vi "Monitoring.vi"() -> ()   [LabVIEW 2014]
uses:
  <vilib>/Instr/_visa.llb/VISA Configure Serial Port (Instr).vi
  Downloads/AttitudeIndicator_lv2012/lv-attitudecontrol.lvlib
panel:
  in  "Tab Control":T1(tab)
  in  "Stop":bool
  in  "Connect":bool
  in  "VISA resource name":refnum<visa-resource-name>="ASRL1::INSTR"
  in  "baud rate":u32=115200
  in  "length of frame":u32=142
  out "error out":errorcluster
  in  "Afficher caractères reçus":bool
  out "received chars":string
  out "Serial Settings:Number of Bytes at Serial Port":u32
  out "Heading":i16
  out "Roll":i16
  out "Pitch":i16
  out "Roll":i16(graph)
  out "Pitch":i16(graph)
  out "Heading":i16(graph)
  in  "Attitude Indicator":refnum<vi>(3d-picture)
  out "Receiver":cluster{u16, u16, u16, u16, u16, u16, u16, u16}(graph)
  out "Ch 0":u16(slide) caption="Gear" scale=0.0..1000.0
  out "Throttle":u16(slide) scale=0.0..1000.0
  out "Roll":u16(slide) scale=0.0..1000.0
  out "Yaw":u16(slide) scale=0.0..1000.0
  out "Pitch":u16(slide) scale=0.0..1000.0
  out "Aux2":u16(slide) scale=0.0..1000.0
  out "Aux1":u16(slide) scale=0.0..1000.0
  out "N/D":u16(slide) scale=0.0..1000.0
  out "Armed":bool
  out "Motors":cluster{u16, u16, u16, u16, u16, u16, u16, u16}(graph)
  out "M 0":u16(slide) scale=0.0..1000.0
  out "M 7":u16(slide) scale=0.0..1000.0
  out "M 6":u16(slide) scale=0.0..1000.0
  out "M 5":u16(slide) scale=0.0..1000.0
  out "M 4":u16(slide) scale=0.0..1000.0
  out "M 3":u16(slide) scale=0.0..1000.0
  out "M 2":u16(slide) scale=0.0..1000.0
  out "M 1":u16(slide) scale=0.0..1000.0
  out "Servos":cluster{u16, u16, u16, u16}(graph)
  out "S 0":u16(slide) scale=0.0..1000.0
  out "S 3":u16(slide) scale=0.0..1000.0
  out "S 2":u16(slide) scale=0.0..1000.0
  out "S 1":u16(slide) scale=0.0..1000.0
  out "Meter":dbl(knob) scale=10800.0..12600.0
  out "Energy":u16
  out "Current":u16
  out "Voltage":u16
  out "Loop duration":u8
  out "Armed":bool
  out "SONAR 0":u16(slide) scale=0.0..1000.0
  out "BARO":u16(slide) scale=0.0..1000.0
  out "SONAR 5":u16(slide) scale=0.0..1000.0
  out "SONAR 4":u16(slide) scale=0.0..1000.0
  out "SONAR 3":u16(slide) scale=0.0..1000.0
  out "SONAR 2":u16(slide) scale=0.0..1000.0
  out "SONAR 1":u16(slide) scale=0.0..1000.0
  out "Baro":u16(graph)
  out "Sonars":cluster{u16, u16, u16, u16, u16, u16}(graph)
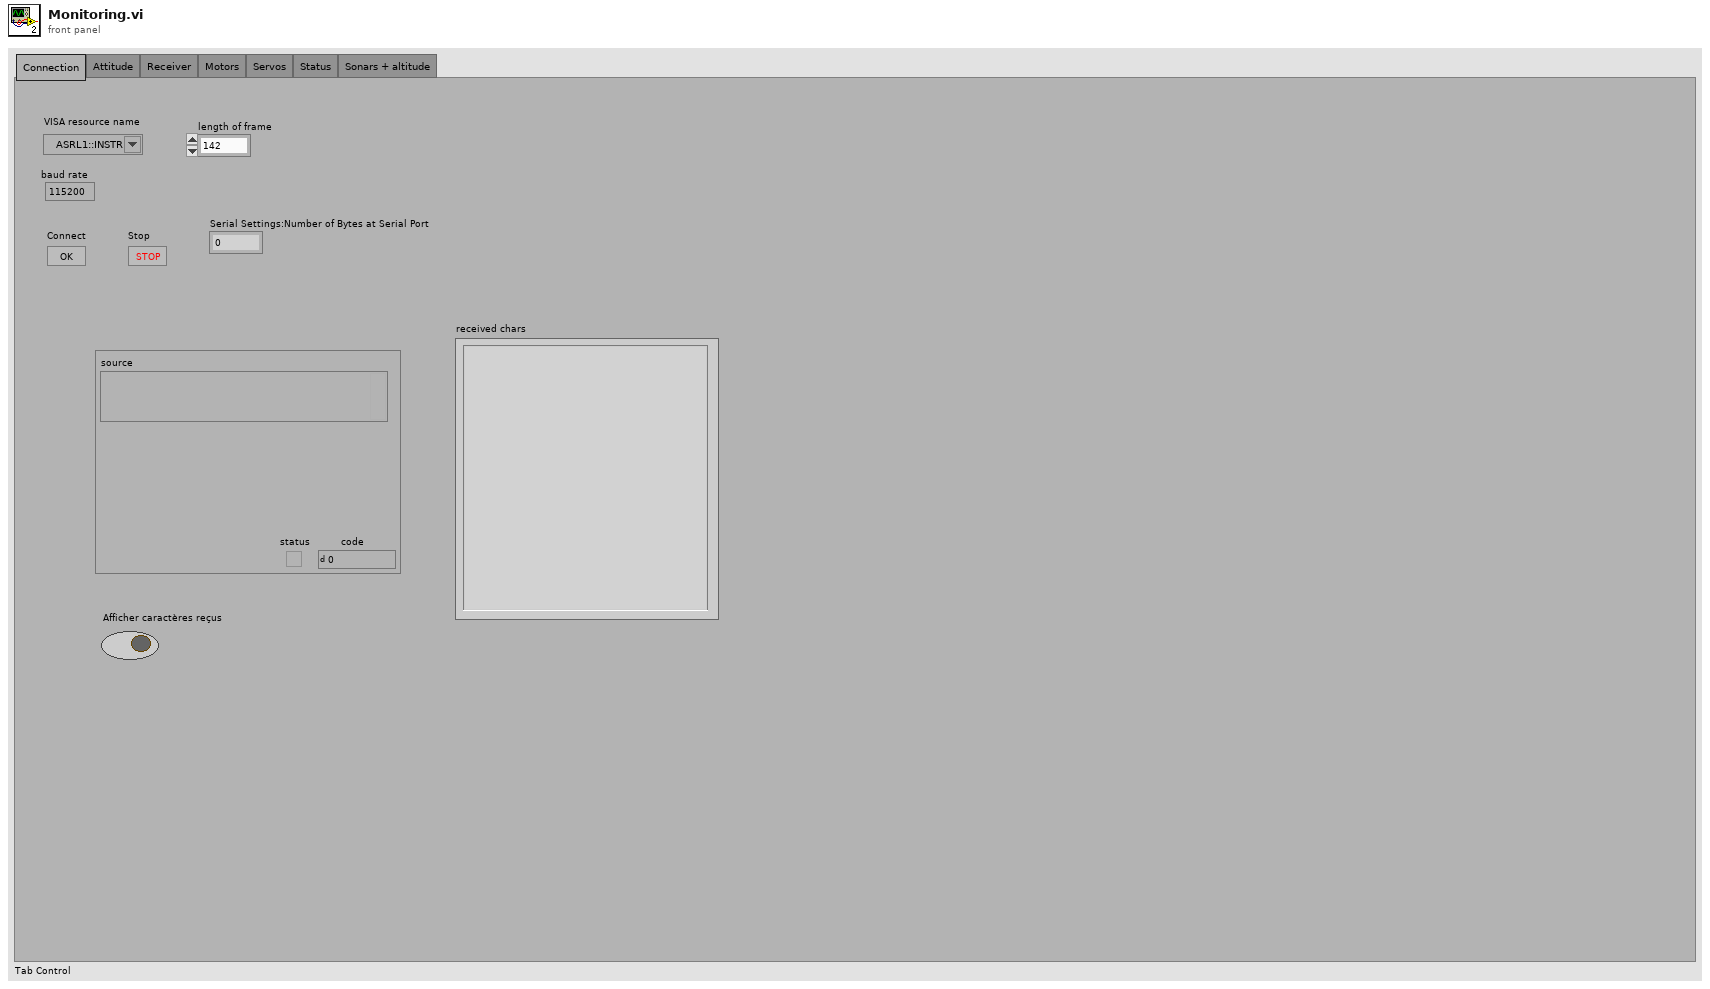
[diagram p1: front panel]
types:
  T1 = enum32{"Connection", "Attitude", "Receiver", "Motors", "Servos", "Status", "Sonars + altitude"}
  T2 = typedef "lv-attitudecontrol.lvlib/AttitudeHandle.ctl" = cluster{"First Scene Object":refnum<vi>, "Drum":refnum<vi>, "Window":refnum<vi>, "Dial":refnum<vi>, "Scene Graph":refnum<vi>, "Last Drum Pitch":dbl, "Last Drum Roll ":dbl, "Last Dial Roll":dbl}
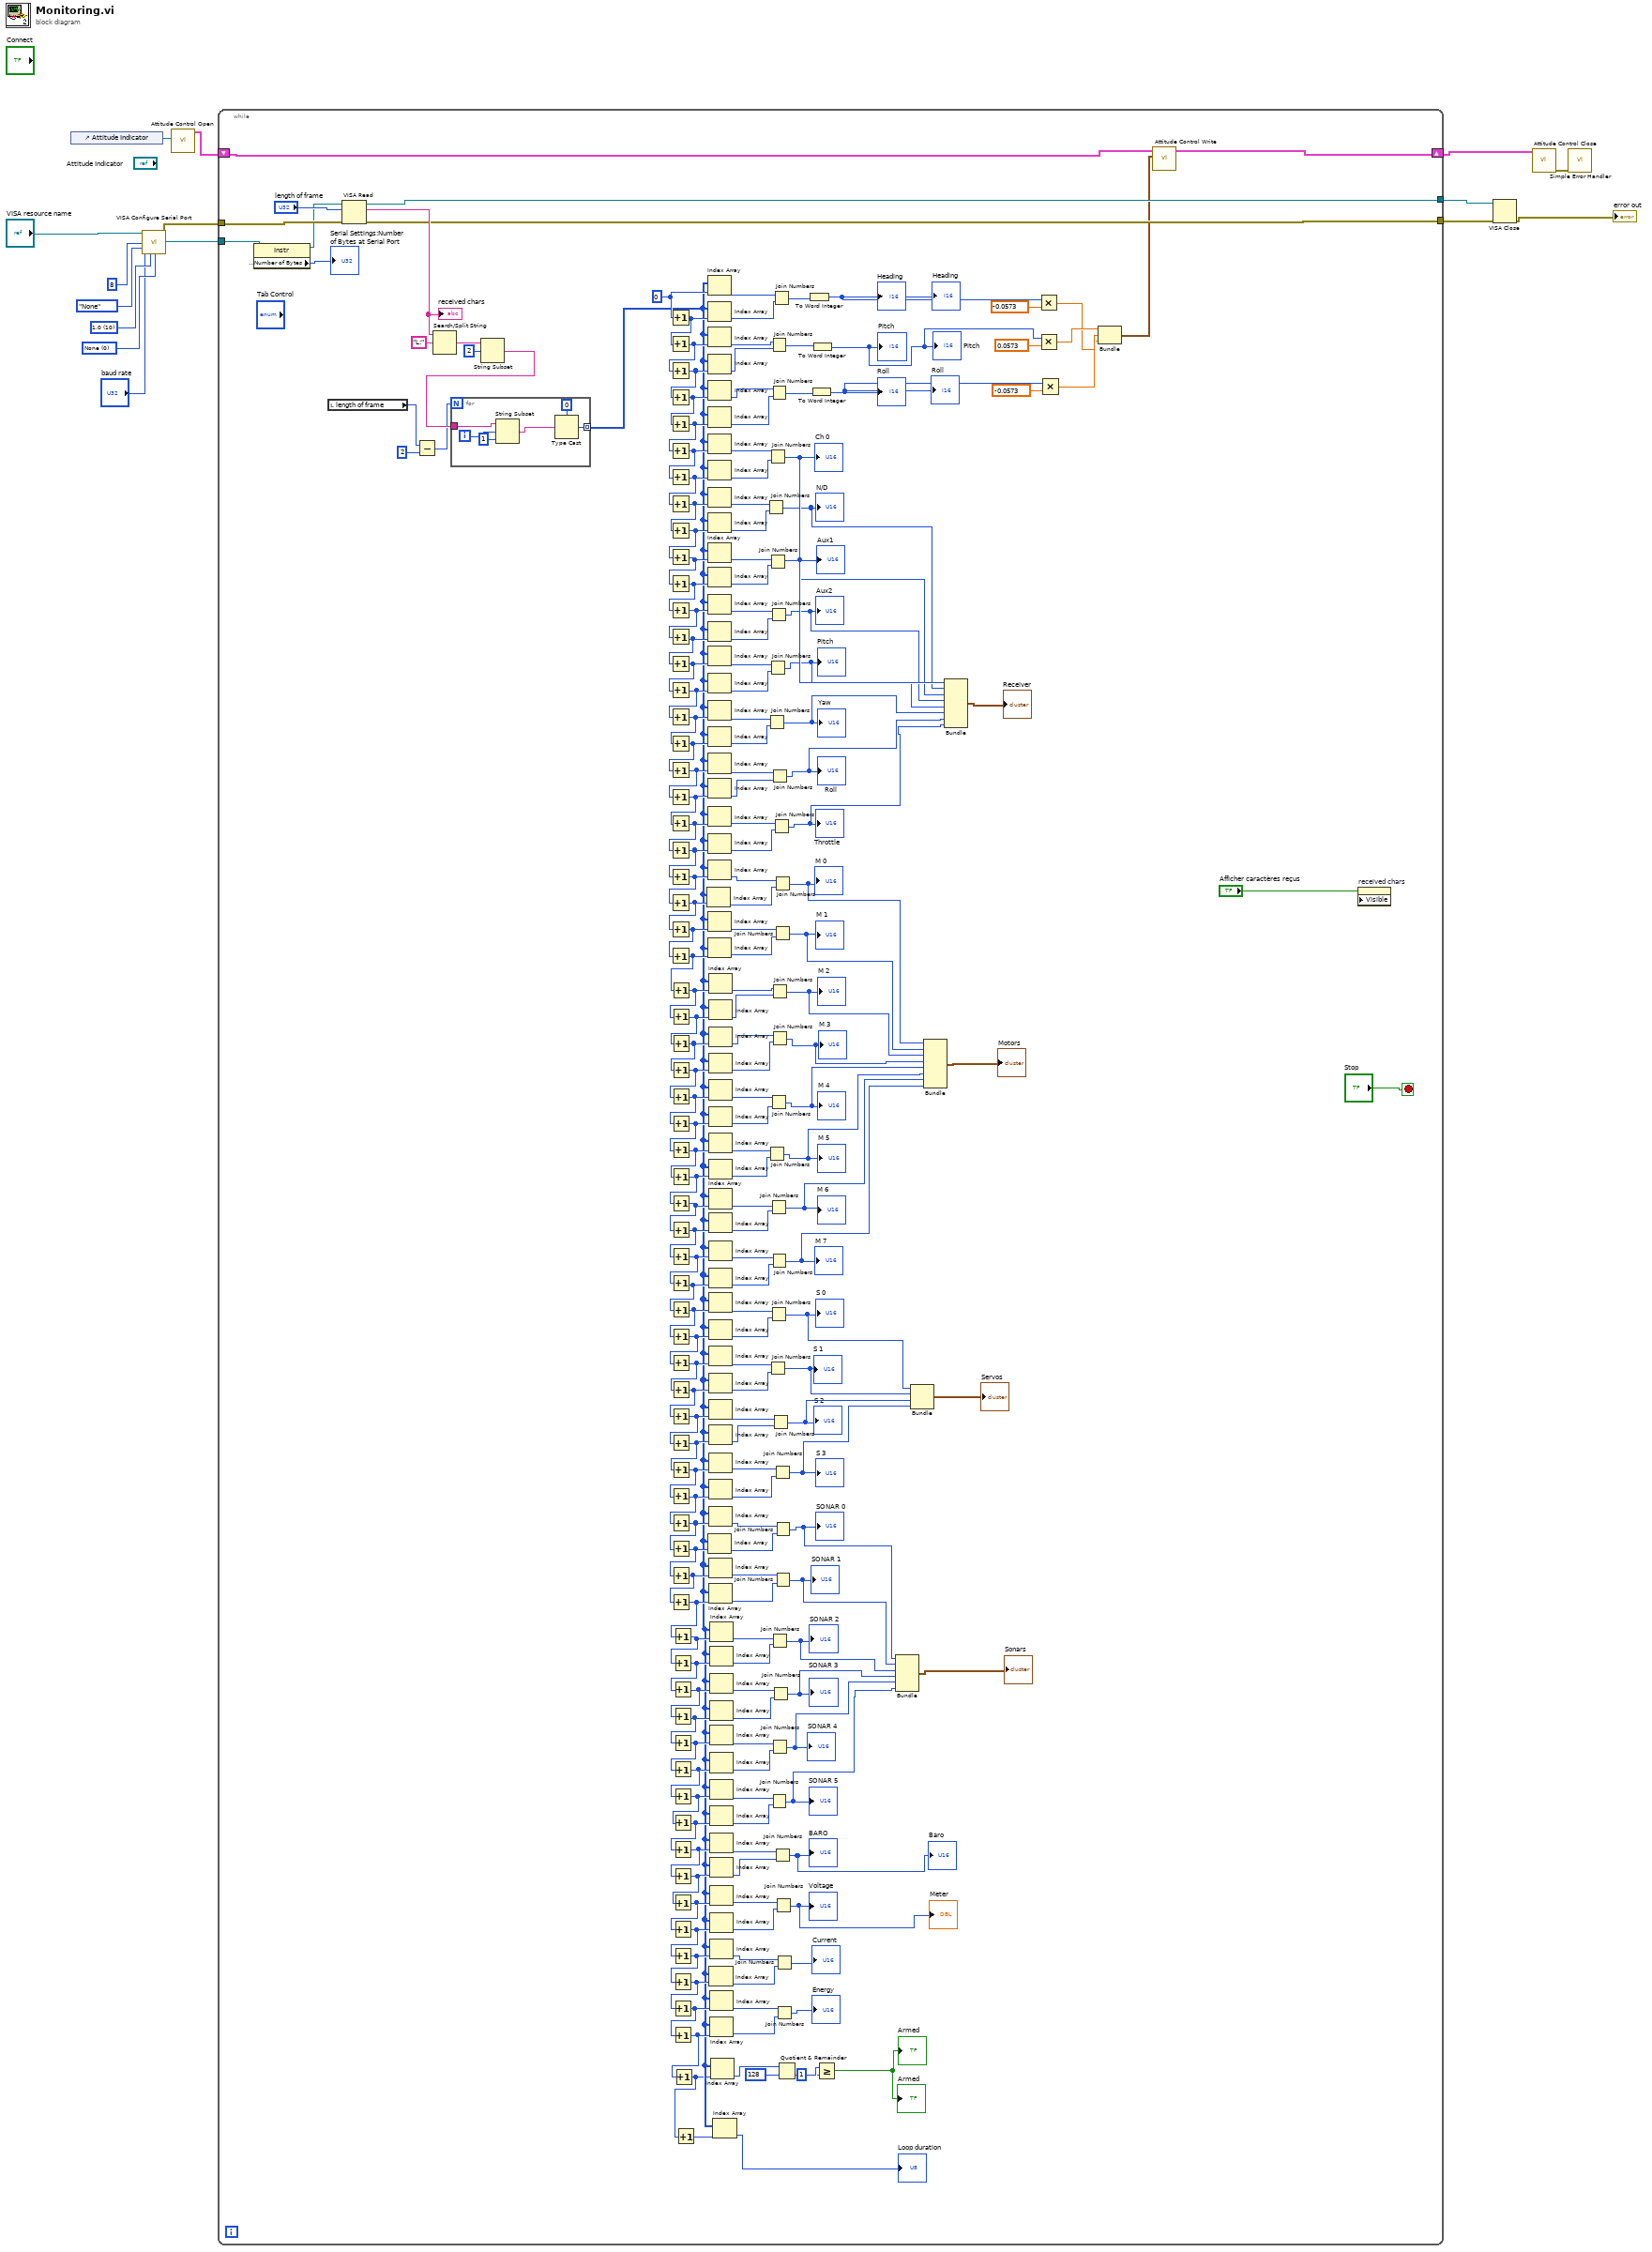
[diagram p0: block diagram]
diagram:
  w12 = u16 0 items=["None", "XON/XOFF", "RTS/CTS", "XON/XOFF & RTS/CTS", "DTR/DSR", "XON/XOFF & DTR/DSR"] ("flow control (0:none)")
  w13 = u16 10 items=["1.0"=10, "1.5"=15, "2.0"=20] ("stop bits (10: 1 bit)")
  n1 = control-ref of="Attitude Indicator"() -> (w4:refnum<vi>)
  n2 = call-poly "VISA Configure Serial Port"("VISA resource name"="VISA resource name", "baud rate (9600)"="baud rate", "data bits (8)"=u16 8, "parity (0:none)"=enum16{"None", "Odd", "Even", "Mark", "Space"}."None", "stop bits (10: 1 bit)"=w13, "flow control (0:none)"=w12) -> ("VISA resource name out"=w10:refnum<visa-resource-name>, "error out"=w9:errorcluster)  [unwired: 8 in]
  n3 = call "Attitude Control Open.vi"("Scene Graph"=w4) -> ("Attitude Control Handle"=w3:T2)  [unwired: 9 in, 1 out]
  n4 = while {
    tunnel: w10 -> [w40]
    tunnel: w9 -> [w192]
    tunnel: [w43] -> w7
    tunnel: [w41] -> w5
    shift-right: [w31] -> w1
    shift-left: w3 -> [w32]
    stop <- "Stop" stop-if-true
    w217 = 0 ("length")
    n5 = property class="Instr"(reference=w40) -> (reference out=w39:refnum<visa-resource-name>, "Serial Settings:Number of Bytes at Serial Port"=→"Serial Settings:Number of Bytes at Serial Port":u32)  [unwired: 1 in, 1 out]
    n6 = local read "length of frame"() -> (w35:u32)
    n7 = VISA Read(VISA resource name=w39, byte count="length of frame", error in (no error)=w192) -> (VISA resource name out=w41:refnum<visa-resource-name>, read buffer=w191:string, error out=w43:errorcluster)  [unwired: 1 out]
    "received chars" <- w191
    n8 = Subtract(x=w35, y=u32 2) -> (x-y=w33:u32)
    n9 = Search/Split String(string=w191, search string/char (-)="L:") -> (match + rest of string=w222:string)  [unwired: 1 in, 2 out]
    n10 = String Subset(string=w222, offset (0)=2) -> (substring=w218:string)  [unwired: 1 in]
    n11 = for {
      N: w33 -> [_]
      tunnel: w218 -> [w225]
      tunnel: [w224] -> w18 mode=indexing
      i -> [w223]
      n12 = String Subset(string=w225, offset (0)=w223, length (rest)=1 ("length (rest)")) -> (substring=w226:string)
      n13 = Type Cast(type=u8 0, x=w226) -> (*(type *) &x=w224:u8)
    }
    n14 = Increment(x=w217) -> (x+1=w216:i32)
    n15 = Increment(x=w216) -> (x+1=w215:i32)
    n16 = Increment(x=w215) -> (x+1=w214:i32)
    n17 = Increment(x=w214) -> (x+1=w213:i32)
    n18 = Increment(x=w213) -> (x+1=w212:i32)
    n19 = Increment(x=w212) -> (x+1=w211:i32)
    n20 = Increment(x=w211) -> (x+1=w210:i32)
    n21 = Increment(x=w210) -> (x+1=w209:i32)
    n22 = Increment(x=w209) -> (x+1=w208:i32)
    n23 = Increment(x=w208) -> (x+1=w207:i32)
    n24 = Increment(x=w207) -> (x+1=w206:i32)
    n25 = Increment(x=w206) -> (x+1=w205:i32)
    n26 = Increment(x=w205) -> (x+1=w204:i32)
    n27 = Increment(x=w204) -> (x+1=w203:i32)
    n28 = Increment(x=w203) -> (x+1=w202:i32)
    n29 = Increment(x=w202) -> (x+1=w201:i32)
    n30 = Increment(x=w201) -> (x+1=w200:i32)
    n31 = Increment(x=w200) -> (x+1=w199:i32)
    n32 = Increment(x=w199) -> (x+1=w198:i32)
    n33 = Increment(x=w198) -> (x+1=w197:i32)
    n34 = Increment(x=w197) -> (x+1=w196:i32)
    n35 = Increment(x=w196) -> (x+1=w195:i32)
    n36 = Increment(x=w195) -> (x+1=w194:i32)
    n37 = Increment(x=w194) -> (x+1=w193:i32)
    n38 = Increment(x=w193) -> (x+1=w115:i32)
    n39 = Increment(x=w115) -> (x+1=w162:i32)
    n40 = Increment(x=w162) -> (x+1=w161:i32)
    n41 = Increment(x=w161) -> (x+1=w160:i32)
    n42 = Increment(x=w160) -> (x+1=w159:i32)
    n43 = Increment(x=w159) -> (x+1=w158:i32)
    n44 = Increment(x=w158) -> (x+1=w157:i32)
    n45 = Increment(x=w157) -> (x+1=w156:i32)
    n46 = Increment(x=w156) -> (x+1=w155:i32)
    n47 = Increment(x=w155) -> (x+1=w154:i32)
    n48 = Increment(x=w154) -> (x+1=w153:i32)
    n49 = Increment(x=w153) -> (x+1=w152:i32)
    n50 = Increment(x=w152) -> (x+1=w151:i32)
    n51 = Increment(x=w151) -> (x+1=w150:i32)
    n52 = Increment(x=w150) -> (x+1=w149:i32)
    n53 = Increment(x=w149) -> (x+1=w148:i32)
    n54 = Increment(x=w148) -> (x+1=w147:i32)
    n55 = Increment(x=w147) -> (x+1=w146:i32)
    n56 = Increment(x=w146) -> (x+1=w145:i32)
    n57 = Increment(x=w145) -> (x+1=w144:i32)
    n58 = Increment(x=w144) -> (x+1=w143:i32)
    n59 = Increment(x=w143) -> (x+1=w142:i32)
    n60 = Increment(x=w142) -> (x+1=w141:i32)
    n61 = Increment(x=w141) -> (x+1=w140:i32)
    n62 = Increment(x=w140) -> (x+1=w83:i32)
    n63 = Increment(x=w83) -> (x+1=w114:i32)
    n64 = Increment(x=w114) -> (x+1=w113:i32)
    n65 = Increment(x=w113) -> (x+1=w112:i32)
    n66 = Increment(x=w112) -> (x+1=w111:i32)
    n67 = Increment(x=w111) -> (x+1=w110:i32)
    n68 = Increment(x=w110) -> (x+1=w109:i32)
    n69 = Increment(x=w109) -> (x+1=w108:i32)
    n70 = Increment(x=w108) -> (x+1=w107:i32)
    n71 = Increment(x=w107) -> (x+1=w106:i32)
    n72 = Increment(x=w106) -> (x+1=w105:i32)
    n73 = Increment(x=w105) -> (x+1=w104:i32)
    n74 = Increment(x=w104) -> (x+1=w103:i32)
    n75 = Increment(x=w103) -> (x+1=w102:i32)
    n76 = Increment(x=w102) -> (x+1=w101:i32)
    n77 = Increment(x=w101) -> (x+1=w100:i32)
    n78 = Increment(x=w100) -> (x+1=w82:i32)
    n79 = Increment(x=w82) -> (x+1=w17:i32)
    n80 = Increment(x=w17) -> (x+1=w19:i32)
    n81 = Index Array(array=w18, index=w194) -> (element=w165:u8)
    n82 = Index Array(array=w18, index=w217) -> (element=w189:u8)
    n83 = Index Array(array=w18, index=w216) -> (element=w190:u8)
    n84 = Index Array(array=w18, index=w215) -> (element=w188:u8)
    n85 = Index Array(array=w18, index=w214) -> (element=w187:u8)
    n86 = Index Array(array=w18, index=w213) -> (element=w186:u8)
    n87 = Index Array(array=w18, index=w212) -> (element=w185:u8)
    n88 = Index Array(array=w18, index=w211) -> (element=w182:u8)
    n89 = Index Array(array=w18, index=w210) -> (element=w181:u8)
    n90 = Index Array(array=w18, index=w209) -> (element=w180:u8)
    n91 = Index Array(array=w18, index=w208) -> (element=w179:u8)
    n92 = Index Array(array=w18, index=w207) -> (element=w178:u8)
    n93 = Index Array(array=w18, index=w206) -> (element=w177:u8)
    n94 = Index Array(array=w18, index=w205) -> (element=w176:u8)
    n95 = Index Array(array=w18, index=w204) -> (element=w175:u8)
    n96 = Index Array(array=w18, index=w203) -> (element=w174:u8)
    n97 = Index Array(array=w18, index=w202) -> (element=w173:u8)
    n98 = Index Array(array=w18, index=w201) -> (element=w172:u8)
    n99 = Index Array(array=w18, index=w200) -> (element=w171:u8)
    n100 = Index Array(array=w18, index=w199) -> (element=w170:u8)
    n101 = Index Array(array=w18, index=w198) -> (element=w169:u8)
    n102 = Index Array(array=w18, index=w197) -> (element=w168:u8)
    n103 = Index Array(array=w18, index=w196) -> (element=w167:u8)
    n104 = Index Array(array=w18, index=w195) -> (element=w166:u8)
    n105 = Index Array(array=w18, index=w193) -> (element=w164:u8)
    n106 = Index Array(array=w18, index=w115) -> (element=w163:u8)
    n107 = Index Array(array=w18, index=w141) -> (element=w118:u8)
    n108 = Index Array(array=w18, index=w162) -> (element=w139:u8)
    n109 = Index Array(array=w18, index=w161) -> (element=w138:u8)
    n110 = Index Array(array=w18, index=w160) -> (element=w137:u8)
    n111 = Index Array(array=w18, index=w159) -> (element=w136:u8)
    n112 = Index Array(array=w18, index=w158) -> (element=w135:u8)
    n113 = Index Array(array=w18, index=w157) -> (element=w134:u8)
    n114 = Index Array(array=w18, index=w156) -> (element=w133:u8)
    n115 = Index Array(array=w18, index=w155) -> (element=w132:u8)
    n116 = Index Array(array=w18, index=w154) -> (element=w131:u8)
    n117 = Index Array(array=w18, index=w153) -> (element=w130:u8)
    n118 = Index Array(array=w18, index=w152) -> (element=w129:u8)
    n119 = Index Array(array=w18, index=w151) -> (element=w128:u8)
    n120 = Index Array(array=w18, index=w150) -> (element=w127:u8)
    n121 = Index Array(array=w18, index=w149) -> (element=w126:u8)
    n122 = Index Array(array=w18, index=w148) -> (element=w125:u8)
    n123 = Index Array(array=w18, index=w147) -> (element=w124:u8)
    n124 = Index Array(array=w18, index=w146) -> (element=w123:u8)
    n125 = Index Array(array=w18, index=w145) -> (element=w122:u8)
    n126 = Index Array(array=w18, index=w144) -> (element=w121:u8)
    n127 = Index Array(array=w18, index=w143) -> (element=w120:u8)
    n128 = Index Array(array=w18, index=w142) -> (element=w119:u8)
    n129 = Index Array(array=w18, index=w140) -> (element=w117:u8)
    n130 = Index Array(array=w18, index=w83) -> (element=w116:u8)
    n131 = Index Array(array=w18, index=w101) -> (element=w86:u8)
    n132 = Index Array(array=w18, index=w114) -> (element=w99:u8)
    n133 = Index Array(array=w18, index=w113) -> (element=w98:u8)
    n134 = Index Array(array=w18, index=w112) -> (element=w97:u8)
    n135 = Index Array(array=w18, index=w111) -> (element=w96:u8)
    n136 = Index Array(array=w18, index=w110) -> (element=w95:u8)
    n137 = Index Array(array=w18, index=w109) -> (element=w94:u8)
    n138 = Index Array(array=w18, index=w108) -> (element=w93:u8)
    n139 = Index Array(array=w18, index=w107) -> (element=w92:u8)
    n140 = Index Array(array=w18, index=w106) -> (element=w91:u8)
    n141 = Index Array(array=w18, index=w105) -> (element=w90:u8)
    n142 = Index Array(array=w18, index=w104) -> (element=w89:u8)
    n143 = Index Array(array=w18, index=w103) -> (element=w88:u8)
    n144 = Index Array(array=w18, index=w102) -> (element=w87:u8)
    n145 = Index Array(array=w18, index=w100) -> (element=w85:u8)
    n146 = Index Array(array=w18, index=w82) -> (element=w84:u8)
    n147 = Index Array(array=w18, index=w17) -> (element=w79:u8)
    n148 = Index Array(array=w18, index=w19) -> (element=→"Loop duration":u8)
    n149 = Join Numbers(hi=w180, lo=w179) -> ((hi.lo)=w73:u16)
    "N/D" <- w73
    n150 = Join Numbers(hi=w172, lo=w171) -> ((hi.lo)=w69:u16)
    "Yaw" <- w69
    n151 = Join Numbers(hi=w133, lo=w132) -> ((hi.lo)=w60:u16)
    "M 5" <- w60
    n152 = Join Numbers(hi=w182, lo=w181) -> ((hi.lo)=w74:u16)
    "Ch 0" <- w74
    n153 = Join Numbers(hi=w178, lo=w177) -> ((hi.lo)=w72:u16)
    "Aux1" <- w72
    n154 = Join Numbers(hi=w174, lo=w173) -> ((hi.lo)=w70:u16)
    "Pitch" <- w70
    n155 = Join Numbers(hi=w125, lo=w124) -> ((hi.lo)=w55:u16)
    "S 1" <- w55
    n156 = Join Numbers(hi=w176, lo=w175) -> ((hi.lo)=w71:u16)
    "Aux2" <- w71
    n157 = Join Numbers(hi=w135, lo=w134) -> ((hi.lo)=w61:u16)
    "M 4" <- w61
    n158 = Join Numbers(hi=w131, lo=w130) -> ((hi.lo)=w59:u16)
    "M 6" <- w59
    n159 = Join Numbers(hi=w127, lo=w126) -> ((hi.lo)=w56:u16)
    "S 0" <- w56
    n160 = Join Numbers(hi=w188, lo=w187) -> ((hi.lo)=w37:u16)
    n161 = Join Numbers(hi=w186, lo=w185) -> ((hi.lo)=w36:u16)
    n162 = Join Numbers(hi=w129, lo=w128) -> ((hi.lo)=w58:u16)
    "M 7" <- w58
    n163 = Join Numbers(hi=w93, lo=w92) -> ((hi.lo)=w45:u16)
    "SONAR 5" <- w45
    n164 = Join Numbers(hi=w170, lo=w169) -> ((hi.lo)=w68:u16)
    "Roll" <- w68
    n165 = Join Numbers(hi=w139, lo=w138) -> ((hi.lo)=w63:u16)
    "M 2" <- w63
    n166 = Join Numbers(hi=w137, lo=w136) -> ((hi.lo)=w62:u16)
    "M 3" <- w62
    n167 = Join Numbers(hi=w99, lo=w98) -> ((hi.lo)=w48:u16)
    "SONAR 2" <- w48
    n168 = Join Numbers(hi=w95, lo=w94) -> ((hi.lo)=w46:u16)
    "SONAR 4" <- w46
    n169 = Join Numbers(hi=w123, lo=w122) -> ((hi.lo)=w54:u16)
    "S 2" <- w54
    n170 = Join Numbers(hi=w97, lo=w96) -> ((hi.lo)=w47:u16)
    "SONAR 3" <- w47
    n171 = Join Numbers(hi=w189, lo=w190) -> ((hi.lo)=w38:u16)
    n172 = Join Numbers(hi=w168, lo=w167) -> ((hi.lo)=w67:u16)
    "Throttle" <- w67
    n173 = Join Numbers(hi=w166, lo=w165) -> ((hi.lo)=w65:u16)
    "M 0" <- w65
    n174 = Join Numbers(hi=w164, lo=w163) -> ((hi.lo)=w64:u16)
    "M 1" <- w64
    n175 = Join Numbers(hi=w121, lo=w120) -> ((hi.lo)=w53:u16)
    "S 3" <- w53
    n176 = Join Numbers(hi=w91, lo=w90) -> ((hi.lo)=→"Baro" →"BARO":u16)
    n177 = Join Numbers(hi=w119, lo=w118) -> ((hi.lo)=w50:u16)
    "SONAR 0" <- w50
    n178 = Join Numbers(hi=w117, lo=w116) -> ((hi.lo)=w49:u16)
    "SONAR 1" <- w49
    n179 = Join Numbers(hi=w89, lo=w88) -> ((hi.lo)=→"Voltage" →"Meter":u16)
    n180 = Join Numbers(hi=w87, lo=w86) -> ((hi.lo)=→"Current":u16)
    n181 = Join Numbers(hi=w85, lo=w84) -> ((hi.lo)=→"Energy":u16)
    n182 = Quotient & Remainder(x=w79, y=u8 128) -> (floor(x/y)=w77:u8)  [unwired: 1 out]
    n183 = To Word Integer(number=w38) -> (16bit integer=w22:i16)
    "Heading" <- w22
    "Heading" <- w22
    n184 = To Word Integer(number=w36) -> (16bit integer=w29:i16)
    "Roll" <- w29
    "Roll" <- w29
    n185 = To Word Integer(number=w37) -> (16bit integer=w21:i16)
    "Pitch" <- w21
    "Pitch" <- w21
    n186 = Greater Or Equal?(x=w77, y=u8 1) -> (x >= y?=→"Armed" →"Armed":bool)
    n187 = Bundle(w50, w49, w48, w47, w46, w45) -> (→"Sonars":cluster{u16, u16, u16, u16, u16, u16})  [unwired: 1 in]
    n188 = Bundle(w56, w55, w54, w53) -> (→"Servos":cluster{u16, u16, u16, u16})  [unwired: 1 in]
    n189 = Bundle(w65, w64, w63, w62, w61, w60, w59, w58) -> (→"Motors":cluster{u16, u16, u16, u16, u16, u16, u16, u16})  [unwired: 1 in]
    n190 = Bundle(w74, w73, w72, w71, w70, w69, w68, w67) -> (→"Receiver":cluster{u16, u16, u16, u16, u16, u16, u16, u16})  [unwired: 1 in]
    n191 = Multiply(x=w22, y=-0.0573) -> (x*y=w26:dbl)
    n192 = Multiply(x=w21, y=0.0573) -> (x*y=w28:dbl)
    n193 = Multiply(x=w29, y=-0.0573) -> (x*y=w27:dbl)
    n194 = Bundle(w28, w27, w26) -> (w25:cluster{dbl, dbl, dbl})  [unwired: 1 in]
    n195 = call "Attitude Control Write.vi"("pitch (x), roll (y), yaw (z)"=w25, "Attitude Control Handle In"=w32) -> ("Attitude Control Handle Out"=w31:T2)  [unwired: 8 in, 1 out]
    n196 = property on="received chars" class="Str"("Visible"="Afficher caractères reçus") -> ()  [unwired: 2 in, 2 out]
  }
  n197 = VISA Close(VISA resource name=w5, error in (no error)=w7) -> (error out=→"error out":errorcluster)
  n198 = call "Attitude Control Close.vi"("Attitude Control Handle"=w1) -> ("error out"=w2:errorcluster)  [unwired: 10 in]
  n199 = call <vilib>:"Simple Error Handler.vi"("error in (no error)"=w2) -> ()  [unwired: 4 in, 5 out]
